vi "Create Object information channels (outgoing).vi"(8 "error in":errorcluster, 11 "Item Ref in":T3 format="%.0x") -> (0 "error out":errorcluster, 3 "Item Ref out":T3 format="%.0x")   [LabVIEW 2019, in "HLA Custom Device System Explorer.lvlib"]
uses:
  HLA Custom Device System Explorer.lvlib
  <vilib>/NI VeriStand/Custom Device API/Custom Device Item Ref.ctl
  emea-ni-adg-hla-lv/src/library/typedefs/TransportationType.ctl
  emea-ni-adg-hla-lv/src/library/typedefs/OrderType.ctl
  <vilib>/NI VeriStand/Custom Device API/Custom Device Channel.ctl
  <vilib>/NI VeriStand/Custom Device API/Custom Device Channel Type.ctl
  <vilib>/NI VeriStand/Custom Device API/Custom Device API.lvlib
  emea-ni-adg-hla-lv/src/library/openrti_rti1516eLv.lvlib
panel:
  in  "OrderType":T1
  in  "TransportType":T2
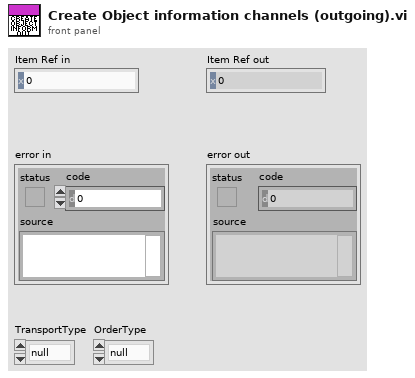
[diagram p1: front panel]
types:
  T1 = typedef "openrti_rti1516eLv.lvlib/OrderType.ctl" = enum32{"null", "RECEIVE", "TIMESTAMP"}
  T2 = typedef "openrti_rti1516eLv.lvlib/TransportationType.ctl" = enum32{"null", "RELIABLE", "BEST_EFFORT"}
  T3 = typedef "Custom Device API.lvlib/Custom Device Item Ref.ctl" = u64
  T4 = typedef "Custom Device API.lvlib/Custom Device Channel.ctl" = cluster{"Type":T5, "Units":string, "Default Value":dbl, "Faultable":bool, "Scalable":bool}
  T5 = typedef "Custom Device API.lvlib/Custom Device Channel Type.ctl" = enum16{"Input", "Output"}
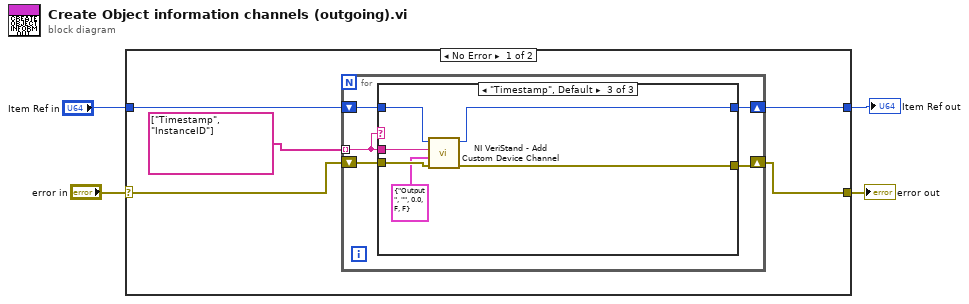
[diagram p0: block diagram]
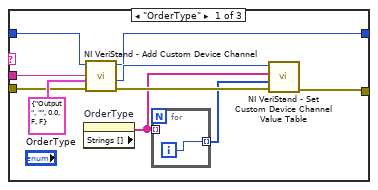
[diagram p2: hidden frame]
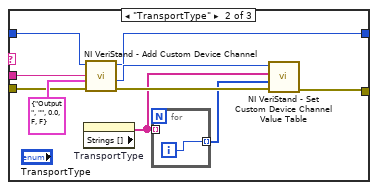
[diagram p3: hidden frame]
diagram:
  n1 = case shown="No Error" "error in" {
    selector: "error in" -> [w7 w43]
    tunnel: [w6 w43] -> w3
    tunnel: [w8 w44] -> w2
    tunnel: "Item Ref in" -> [w9 w44]
    frame No Error {
      n2 = for {
        shift-right: [w13] -> w8
        shift-left: w9 -> [w14]
        shift-right: [w11] -> w6
        shift-left: w7 -> [w12]
        tunnel: string[] ["Timestamp", "InstanceID"] -> [w10] mode=indexing
        n3 = case shown="\"Timestamp\", Default" w10 {
          tunnel: w14 -> [w21 w32 w42]
          tunnel: [w17 w28 w41] -> w13
          tunnel: w12 -> [w23 w34 w40]
          tunnel: [w19 w30 w39] -> w11
          tunnel: w10 -> [w22 w33 w38]
          frame "OrderType" {
            n4 = property on="OrderType" class="Enum (strict)"() -> ("Strings []"=w16:string[])  [unwired: 2 in, 2 out]
            n5 = call <vilib>:"NI VeriStand - Add Custom Device Channel.vi"("error in (no error)"=w23, "Channel"=T4 {"Type"=enum."Output", "Units"="", "Default Value"=0.0, "Faultable"=FALSE, "Scalable"=FALSE}, "Channel Name"=w22, "Parent Ref in"=w21) -> ("error out"=w20:errorcluster, "Channel Ref"=w18:T3, "Parent Ref out"=w17:T3)  [unwired: 4 in, 1 out]
            n6 = for {
              tunnel: w16 -> [_] mode=indexing
              tunnel: [w25] -> w15 mode=indexing
              i -> [w25]
            }
            n7 = call <vilib>:"NI VeriStand - Set Custom Device Channel Value Table.vi"("error in (no error)"=w20, "Values"=w15, "Names"=w16, "Channel Ref in"=w18) -> ("error out"=w19:errorcluster)  [unwired: 6 in, 1 out]
          }
          frame "TransportType" {
            n8 = property on="TransportType" class="Enum (strict)"() -> ("Strings []"=w27:string[])  [unwired: 2 in, 2 out]
            n9 = call <vilib>:"NI VeriStand - Add Custom Device Channel.vi"("error in (no error)"=w34, "Channel"=T4 {"Type"=enum."Output", "Units"="", "Default Value"=0.0, "Faultable"=FALSE, "Scalable"=FALSE}, "Channel Name"=w33, "Parent Ref in"=w32) -> ("error out"=w31:errorcluster, "Channel Ref"=w29:T3, "Parent Ref out"=w28:T3)  [unwired: 4 in, 1 out]
            n10 = for {
              tunnel: w27 -> [_] mode=indexing
              tunnel: [w36] -> w26 mode=indexing
              i -> [w36]
            }
            n11 = call <vilib>:"NI VeriStand - Set Custom Device Channel Value Table.vi"("error in (no error)"=w31, "Values"=w26, "Names"=w27, "Channel Ref in"=w29) -> ("error out"=w30:errorcluster)  [unwired: 6 in, 1 out]
          }
          frame "Timestamp", Default {
            n12 = call <vilib>:"NI VeriStand - Add Custom Device Channel.vi"("error in (no error)"=w40, "Channel"=T4 {"Type"=enum."Output", "Units"="", "Default Value"=0.0, "Faultable"=FALSE, "Scalable"=FALSE}, "Channel Name"=w38, "Parent Ref in"=w42) -> ("error out"=w39:errorcluster, "Parent Ref out"=w41:T3)  [unwired: 4 in, 2 out]
          }
        }
      }
    }
    frame Error {
    }
  }
  "error out" <- w3
  "Item Ref out" <- w2
